vi "ReadMathcadValues.vi"(10 "Name.Sub":string[](array[string]), 11 "Regions":string[](array[string])) -> (3 "Variable Clusters out":T1)   [LabVIEW 2012, in "Design Server.lvlib"]
uses:
  Design Server.lvlib
  Variable cluster.ctl
panel:
  out "Array":string[](array[string])
  out "error IO":errorcluster
  in  "error in":errorcluster
  out "Numeric":i32
  in  "Variable Clusters":T1
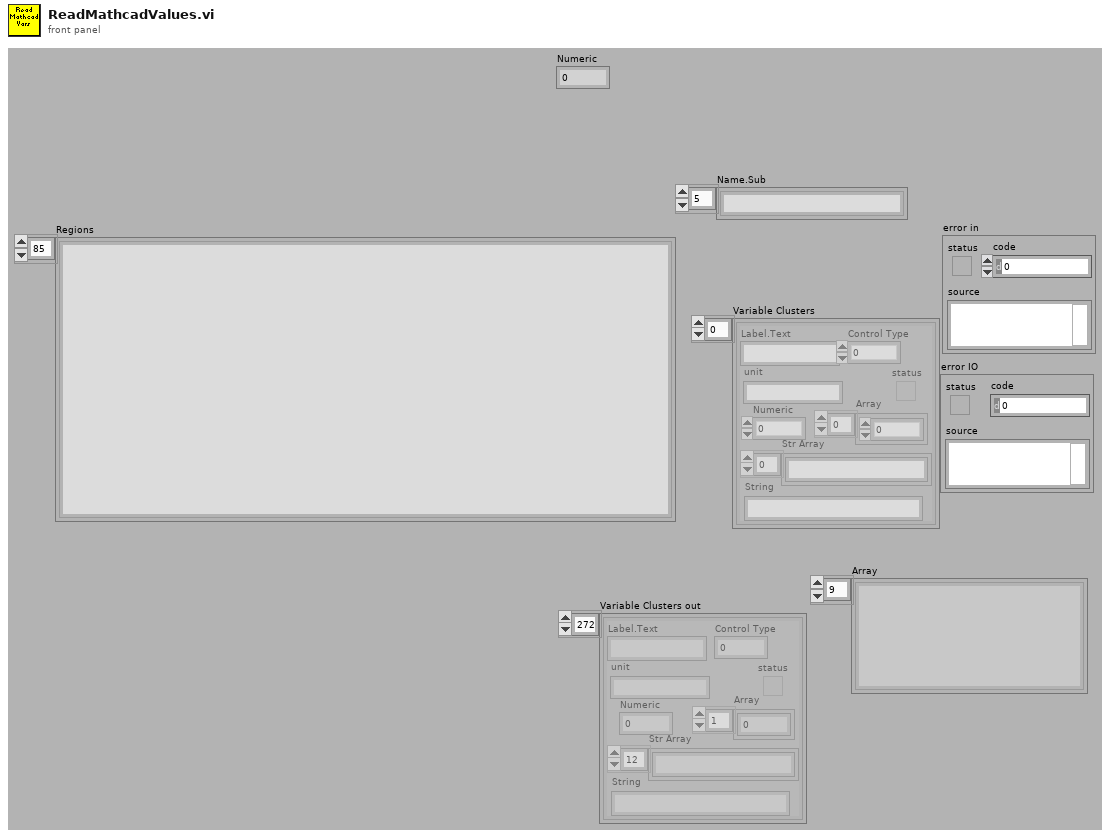
[diagram p1: front panel]
types:
  T1 = typedef "Design Server.lvlib/Variable cluster.ctl" = cluster{"Label.Text":string, "Control Type":u32, "Numeric":dbl, "Array":dbl[], "status":bool, "Str Array":string[], "String":string, "unit":string}[]
  T2 = cluster{"Label.Text":string, "Control Type":u32, "Numeric":dbl, "Array":dbl[], "status":bool, "Str Array":string[], "String":string, "unit":string}
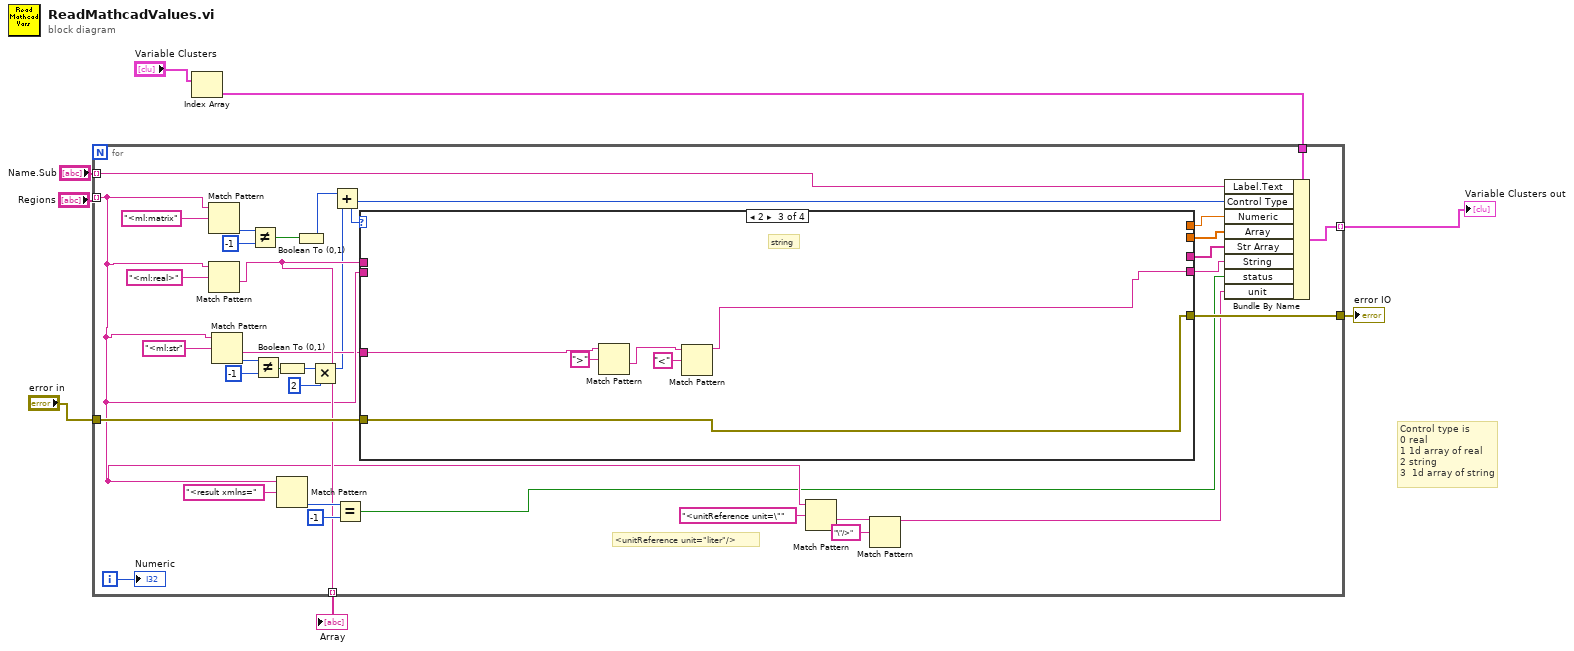
[diagram p0: block diagram]
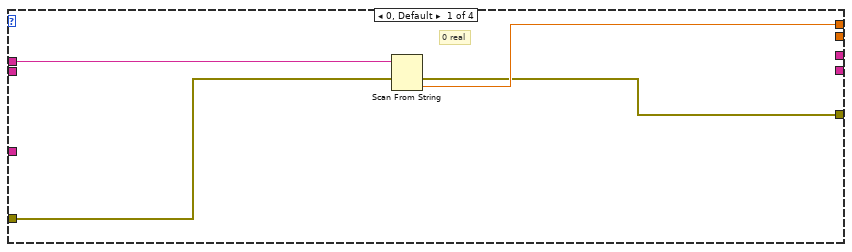
[diagram p2: hidden frame]
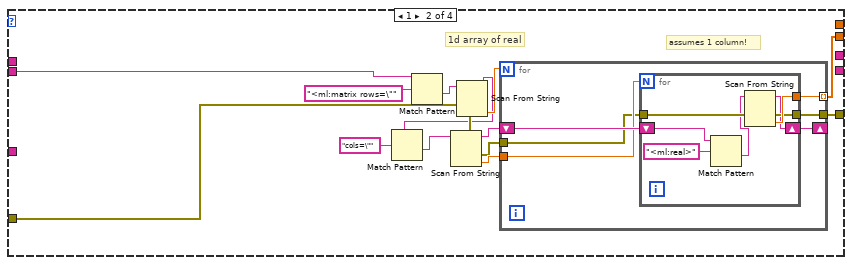
[diagram p3: hidden frame]
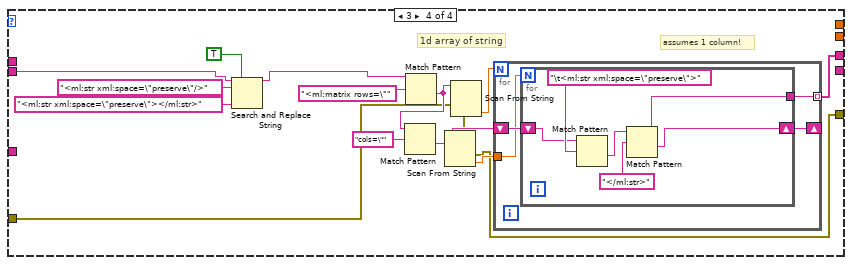
[diagram p4: hidden frame]
diagram:
  # "Control type is\n0 real\n1 1d array of real\n2 string\n3  1d array of string"
  n1 = Index Array(array="Variable Clusters") -> (element=w5:T2)  [unwired: 1 in]
  n2 = for {
    tunnel: "Regions" -> [w18] mode=indexing
    tunnel: "Name.Sub" -> [w41] mode=indexing
    tunnel: w5 -> [w43]
    tunnel: [w42] -> w4 mode=indexing
    tunnel: "error in" -> [w21]
    tunnel: [w20] -> w2
    tunnel: [w19] -> w1 mode=indexing
    i -> [w22]
    # "<unitReference unit=\"liter\"/>"
    n3 = Match Pattern(string=w18, regular expression="<ml:matrix") -> (offset past match=w36:i32)  [unwired: 1 in, 3 out]
    n4 = Match Pattern(string=w18, regular expression="<ml:real>") -> (after substring=w19:string)  [unwired: 1 in, 3 out]
    n5 = Match Pattern(string=w18, regular expression="<ml:str") -> (after substring=w13:string, offset past match=w32:i32)  [unwired: 1 in, 2 out]
    n6 = Not Equal?(x=w36, y=-1) -> (x != y?=w30:bool)
    n7 = Not Equal?(x=w32, y=-1) -> (x != y?=w28:bool)
    n8 = Boolean To (0,1)(Boolean=w28) -> (0, 1=w27:i16)
    n9 = Match Pattern(string=w18, regular expression="<result xmlns=") -> (offset past match=w39:i32)  [unwired: 1 in, 3 out]
    n10 = Boolean To (0,1)(Boolean=w30) -> (0, 1=w29:i16)
    n11 = Multiply(x=w27, y=i16 2) -> (x*y=w10:i16)
    n12 = Add(x=w29, y=w10) -> (x+y=w26:i16)
    n13 = Equal?(x=w39, y=-1) -> (x = y?=w12:bool)
    n14 = case shown="2" w26 {
      tunnel: w18 -> [_ w61 _ w85]
      tunnel: w19 -> [w47 _ _ _]
      tunnel: [w46 _ _ _] -> w25
      tunnel: [_ w58 _ _] -> w24
      tunnel: [_ _ _ w93] -> w23
      tunnel: w21 -> [w45 w55 w80 w88]
      tunnel: [w44 w52 w80 w86] -> w20
      tunnel: w13 -> [_ _ w76 _]
      tunnel: [_ _ w75 _] -> w11
      frame 0, Default {
        # "0 real"
        n15 = Scan From String(input string=w47, error in=w45) -> (error out=w44:errorcluster, output 1=w46:dbl)  [unwired: 3 in, 2 out]
      }
      frame 1 {
        # "assumes 1 column!"
        # "1d array of real"
        n16 = Match Pattern(string=w61, regular expression="<ml:matrix rows=\"") -> (after substring=w51:string)  [unwired: 1 in, 3 out]
        n17 = Scan From String(input string=w51, error in=w55) -> (remaining string=w50:string, error out=w54:errorcluster, output 1=w56:dbl)  [unwired: 3 in, 1 out]
        n18 = Match Pattern(string=w50, regular expression="cols=\"") -> (after substring=w49:string)  [unwired: 1 in, 3 out]
        n19 = Scan From String(input string=w49, error in=w54) -> (remaining string=w48:string, error out=w53:errorcluster, output 1=w57:dbl)  [unwired: 3 in, 1 out]
        n20 = for {
          N: w56 -> [_]
          shift-right: [w67] -> _
          shift-left: w48 -> [w66]
          tunnel: w57 -> [w65]
          tunnel: [w64] -> w58 mode=indexing
          tunnel: w53 -> [w63]
          tunnel: [w62] -> w52
          n21 = for {
            N: w65 -> [_]
            shift-right: [w69] -> w67
            shift-left: w66 -> [w73]
            tunnel: [w72] -> w64
            tunnel: w63 -> [w71]
            tunnel: [w70] -> w62
            n22 = Match Pattern(string=w73, regular expression="<ml:real>") -> (after substring=w68:string)  [unwired: 1 in, 3 out]
            n23 = Scan From String(input string=w68, error in=w71) -> (remaining string=w69:string, error out=w70:errorcluster, output 1=w72:dbl)  [unwired: 3 in, 1 out]
          }
        }
      }
      frame 2 {
        # "string"
        n24 = Match Pattern(string=w76, regular expression=">") -> (after substring=w77:string)  [unwired: 1 in, 3 out]
        n25 = Match Pattern(string=w77, regular expression="<") -> (before substring=w75:string)  [unwired: 1 in, 3 out]
      }
      frame 3 {
        # "assumes 1 column!"
        # "1d array of string"
        n26 = Search and Replace String(replace all?=TRUE ("replace all? (F)"), input string=w85, search string="<ml:str xml:space=\"preserve\"/>", replace string="<ml:str xml:space=\"preserve\"></ml:str>" ("replace string (\"\")")) -> (result string=w84:string)  [unwired: 4 in, 3 out]
        n27 = Match Pattern(string=w84, regular expression="<ml:matrix rows=\"") -> (after substring=w90:string)  [unwired: 1 in, 3 out]
        n28 = Match Pattern(string=w90, regular expression="cols=\"") -> (after substring=w89:string)  [unwired: 1 in, 3 out]
        n29 = Scan From String(input string=w90, error in=w88) -> (error out=w87:errorcluster, output 1=w92:dbl)  [unwired: 3 in, 2 out]
        n30 = Scan From String(input string=w89, error in=w87) -> (error out=w86:errorcluster, output 1=w91:dbl)  [unwired: 3 in, 2 out]
        n31 = for {
          N: w92 -> [_]
          shift-right: [w99] -> _
          shift-left: w89 -> [w98]
          tunnel: w91 -> [w97]
          tunnel: [w96] -> w93 mode=indexing
          n32 = for {
            N: w97 -> [_]
            shift-right: [w100] -> w99
            shift-left: w98 -> [w104]
            tunnel: [w103] -> w96
            n33 = Match Pattern(string=w104, regular expression="\t<ml:str xml:space=\"preserve\">") -> (after substring=w102:string)  [unwired: 1 in, 3 out]
            n34 = Match Pattern(string=w102, regular expression="</ml:str>") -> (before substring=w103:string, after substring=w100:string)  [unwired: 1 in, 2 out]
          }
        }
      }
    }
    n35 = Match Pattern(string=w18, regular expression="<unitReference unit=\"") -> (after substring=w16:string)  [unwired: 1 in, 3 out]
    n36 = Match Pattern(string=w16, regular expression="\"/>") -> (before substring=w14:string)  [unwired: 1 in, 3 out]
    n37 = Bundle By Name(cluster=w43, "Label.Text"=w41, "Control Type"=w26, "Numeric"=w25, "Array"=w24, "Str Array"=w23, "String"=w11, "status"=w12, "unit"=w14) -> (w42:T2)
    "Numeric" <- w22
  }
  "Variable Clusters out" <- w4
  "error IO" <- w2
  "Array" <- w1
